vi "opencvSegmentMultiple.vi"(6 "maxYInStack":dbl, 7 "maxXInStack":dbl, 8 "ImgIn":u16[][][](array[numeric])) -> (0 "NeuronN[last frame]":u16, 1 "maxY":dbl, 2 "NeuronXY[last frame]":u16[](array[numeric]), 3 "NeuronN[frame]":u16[](array[numeric]), 4 "maxX":dbl, 5 "NeuronXY[frame]":u16[][](array[numeric]))   [LabVIEW 2017]
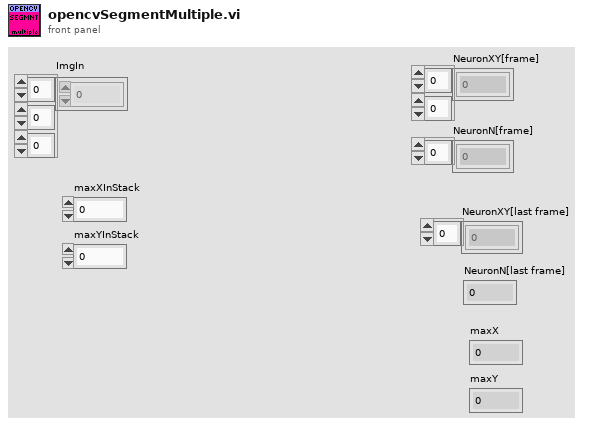
[diagram p1: front panel]
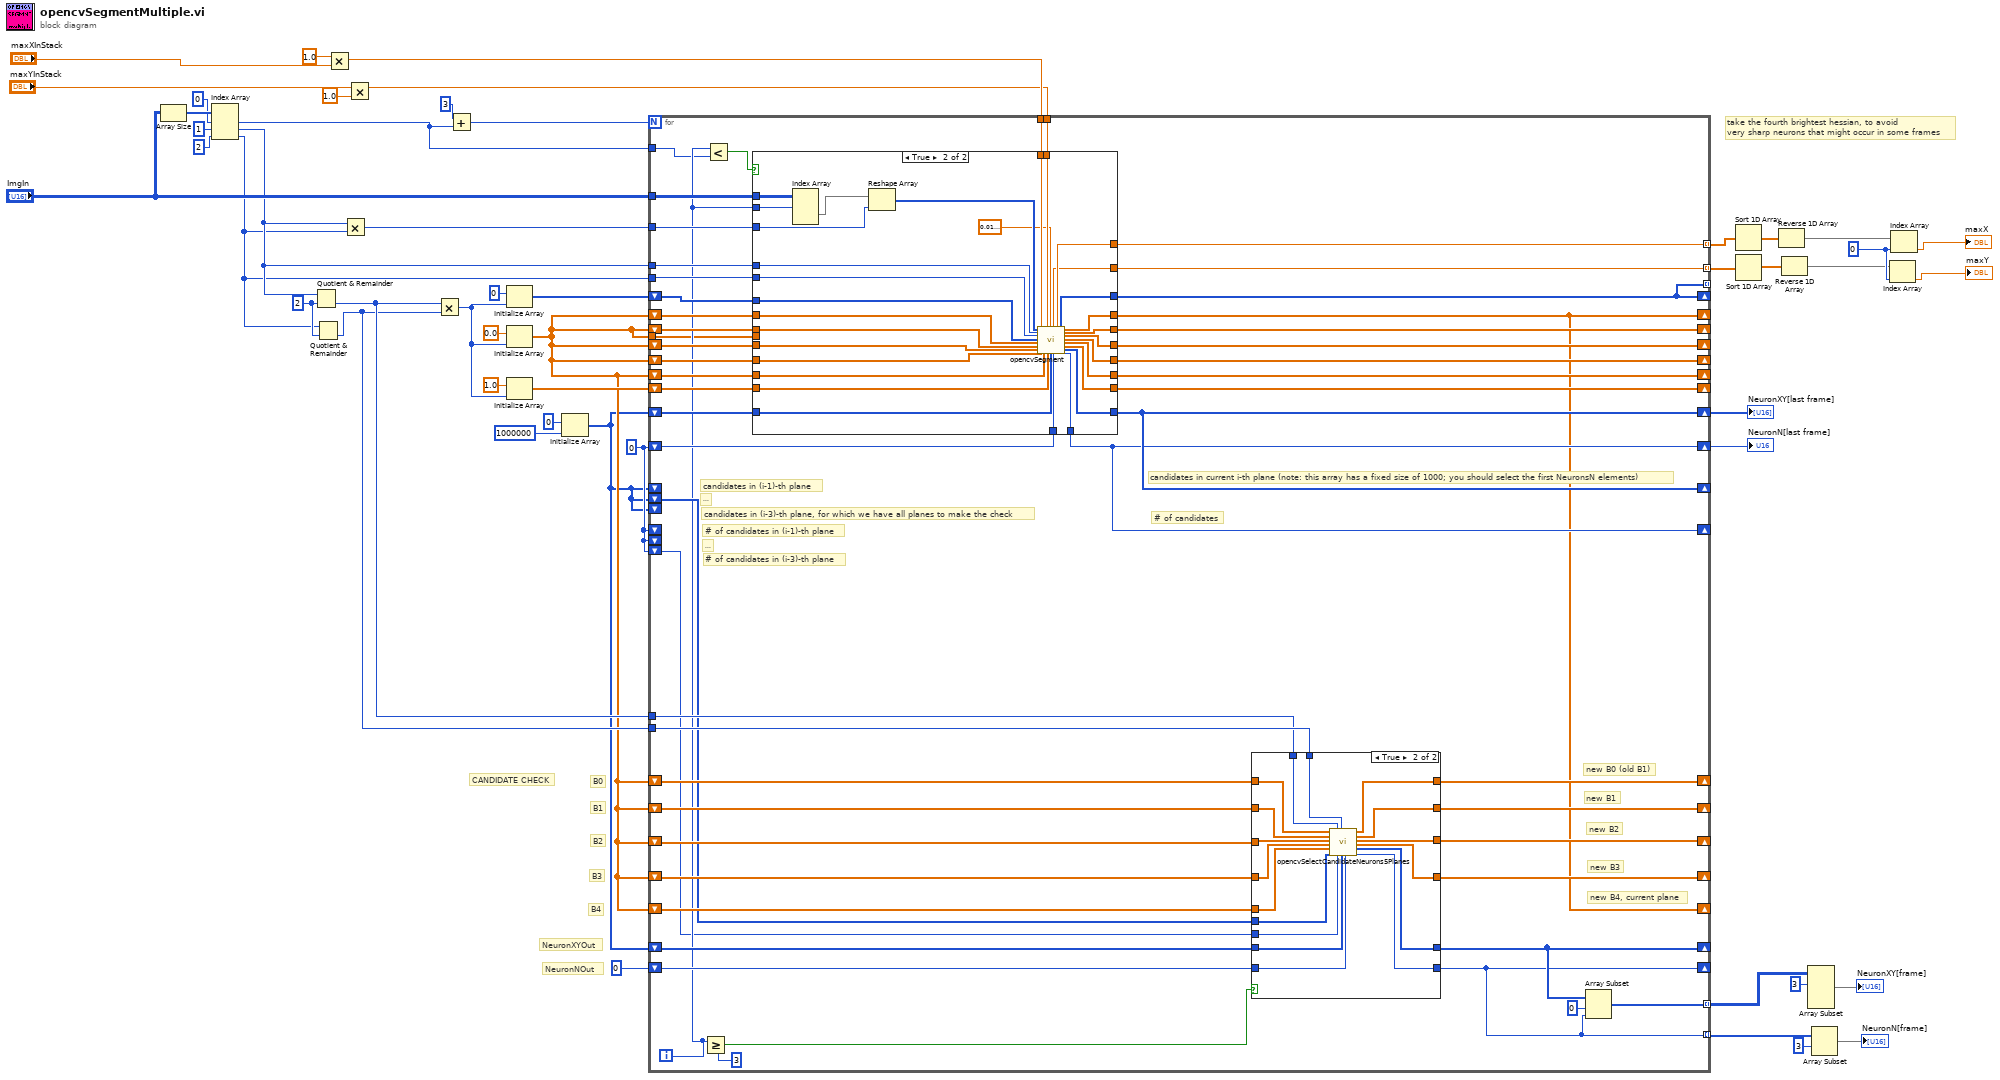
[diagram p0: block diagram]
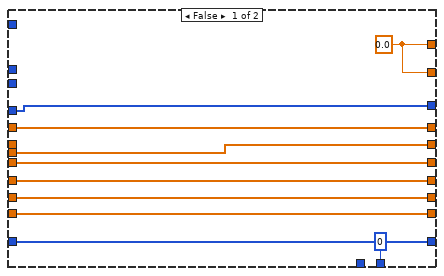
[diagram p2: hidden frame]
diagram:
  w3 = 0 ("y")
  w37 = 2 ("y")
  w11 = u16 0
  # "take the fourth brightest hessian, to avoid\nvery sharp neurons that might occur in some frames"
  # "NeuronNOut"
  # "NeuronXYOut"
  # "B4"
  # "B3"
  # "B2"
  # "B1"
  # "B0"
  # "CANDIDATE CHECK"
  n1 = Array Size(array="ImgIn") -> (size(s)=w49:i32[])
  n2 = Index Array(array=w49, index #1=0 ("index"), index #2=1 ("index"), index #3=2 ("index")) -> (element #1=w6:i32, element #2=w35:i32, element #3=w34:i32)
  n3 = Quotient & Remainder(x=w35, y=w37) -> (floor(x/y)=w32:i32)  [unwired: 1 out]
  n4 = Quotient & Remainder(x=w34, y=w37) -> (floor(x/y)=w31:i32)  [unwired: 1 out]
  n5 = Multiply(x=1.0, y="maxXInStack") -> (x*y=w25:dbl)
  n6 = Multiply(x=w35, y=w34) -> (x*y=w33:i32)
  n7 = Multiply(x="maxYInStack", y=1.0) -> (x*y=w23:dbl)
  n8 = Multiply(x=w32, y=w31) -> (x*y=w36:i32)
  n9 = Add(x=3, y=w6) -> (x+y=w18:i32)
  n10 = Initialize Array(u16 0 ("element"), w36) -> (w43:u16[])
  n11 = Initialize Array(sgl 0.0 ("element"), w36) -> (w13:sgl[])
  n12 = Initialize Array(sgl 1.0 ("element"), w36) -> (w42:sgl[])
  n13 = Initialize Array(u16 0 ("element"), 1000000 ("dimension size")) -> (w10:u16[])
  n14 = for {
    N: w18 -> [_]
    tunnel: "ImgIn" -> [w60]
    shift-right: [w50] -> _
    shift-left: w43 -> [w98]
    shift-right: [w52] -> _
    shift-left: w13 -> [w97]
    shift-right: [w53] -> _
    shift-left: w13 -> [w96]
    shift-right: [w63] -> _
    shift-left: w13 -> [w95]
    shift-right: [w62] -> _
    shift-left: w13 -> [w94]
    shift-right: [w61] -> _
    shift-left: w13 -> [w93]
    shift-right: [w88] -> _
    shift-left: w42 -> [w92]
    shift-right: [w72] -> w29
    shift-left: w10 -> [w91]
    shift-right: [w64] -> w28
    shift-left: w11 -> [w90]
    tunnel: w33 -> [w89]
    tunnel: w35 -> [w100]
    tunnel: w34 -> [w99]
    shift-right: [w77] -> _
    shift-left: w13 -> [w86]
    shift-right: [w76] -> _
    shift-left: w13 -> [w85]
    shift-right: [w75] -> _
    shift-left: w13 -> [w84]
    shift-right: [w74] -> _
    shift-left: w13 -> [w83]
    shift-right: [w52] -> _
    shift-left: w13 -> [w82]
    tunnel: w32 -> [w80]
    tunnel: w31 -> [w81]
    shift-right: [w73] -> _
    shift-left: w10 -> [w79]
    shift-right: [w55] -> _
    shift-left: u16 0 -> [w78]
    shift-right: [w72] -> _
    shift-left: w10 -> [_]
    shift-right: [w64] -> _
    shift-left: w11 -> [_]
    shift-left: w10 -> [w71]
    shift-left: w11 -> [_]
    tunnel: [w69] -> w9 mode=indexing
    tunnel: [w55] -> w16 mode=indexing
    tunnel: w25 -> [w68]
    tunnel: w23 -> [w67]
    tunnel: [w66] -> w21 mode=indexing
    tunnel: [w65] -> w7 mode=indexing
    tunnel: w6 -> [w58]
    tunnel: w13 -> [w54]
    shift-left: w11 -> [w51]
    shift-left: w10 -> [_]
    tunnel: [w50] -> _ mode=indexing
    i -> [w59]
    # "candidates in (i-3)-th plane, for which we have all planes to make the check"
    # "# of candidates in (i-3)-th plane"
    # "..."
    # "# of candidates in (i-1)-th plane"
    # "new B4, current plane"
    # "new B3"
    # "new B2"
    # "new B1"
    # "new B0 (old B1)"
    # "# of candidates"
    # "..."
    # "candidates in (i-1)-th plane"
    # "candidates in current i-th plane (note: this array has a fixed size of 1000; you should select the first NeuronsN elements)"
    n15 = Greater Or Equal?(x=w59, y=3) -> (x >= y?=w56:bool)
    n16 = Less?(x=w59, y=w58) -> (x < y?=w57:bool)
    n17 = case shown="True" w57 {
      tunnel: w100 -> [_ w140]
      tunnel: w99 -> [_ w139]
      tunnel: w98 -> [w109 w138]
      tunnel: w97 -> [w108 w137]
      tunnel: w96 -> [_ w136]
      tunnel: w95 -> [w107 w135]
      tunnel: w94 -> [w106 w134]
      tunnel: w93 -> [w105 w133]
      tunnel: w92 -> [w104 w132]
      tunnel: w91 -> [w103 w131]
      tunnel: w90 -> [_ w130]
      tunnel: w89 -> [_ w129]
      tunnel: [w104 w128] -> w88
      tunnel: [w103 w127] -> w72
      tunnel: w68 -> [_ w125]
      tunnel: w67 -> [_ w124]
      tunnel: [w110 w123] -> w66
      tunnel: [w110 w122] -> w65
      tunnel: [u16 0 ("NeuronN Out") w121] -> w64
      tunnel: [w101 w120] -> w53
      tunnel: [w107 w119] -> w63
      tunnel: [w106 w118] -> w62
      tunnel: [w105 w117] -> w61
      tunnel: [w109 w116] -> w50
      tunnel: [w108 w115] -> w52
      tunnel: w60 -> [_ w114]
      tunnel: w59 -> [_ w112]
      tunnel: w54 -> [w101 _]
      frame False {
        w110 = 0.0 ("maxX")
      }
      frame True {
        n18 = Index Array(array=w114, index (dim 0)=w112) -> (element=w113:u16[][])  [unwired: 2 in]
        n19 = Reshape Array(w113, w129) -> (w126:u16[])
        n20 = call "opencvSegment.vi"("ImgIn"=w126, "sizex"=w140, "sizey"=w139, "ArrA"=w138, "ArrB"=w137, "ArrBX"=w136, "ArrBY"=w135, "ArrBth"=w134, "maxXInStack"=w125, "ArrBdil"=w133, "maxYInStack"=w124, "ArrUno"=w132, "threshold"=sgl 0.02, "NeuronXY"=w131, "NeuronN"=w130) -> ("maxY"=w122:dbl, "maxX"=w123:dbl, "ArrA Out"=w116:u16[], "ArrB Out"=w115:sgl[], "ArrBX Out"=w120:sgl[], "ArrBY Out"=w119:sgl[], "ArrBth Out"=w118:sgl[], "ArrBdil Out"=w117:sgl[], "ArrUno Out"=w128:sgl[], "NeuronXY Out"=w127:u16[], "NeuronN Out"=w121:u16)  [unwired: 2 in]
      }
    }
    n21 = case shown="True" w56 {
      tunnel: w86 -> [_ w163]
      tunnel: w85 -> [w146 w162]
      tunnel: w84 -> [w145 w161]
      tunnel: w83 -> [w144 w160]
      tunnel: w82 -> [w143 w159]
      tunnel: w81 -> [_ w147]
      tunnel: w80 -> [_ w158]
      tunnel: w79 -> [w142 w157]
      tunnel: w78 -> [w141 w156]
      tunnel: [w146 w155] -> w77
      tunnel: [w145 w154] -> w76
      tunnel: [w144 w153] -> w75
      tunnel: [w143 w152] -> w74
      tunnel: [w142 w151] -> w73
      tunnel: [w141 w150] -> w55
      tunnel: w51 -> [_ w149]
      tunnel: w71 -> [_ w148]
      frame False {
      }
      frame True {
        n22 = call "opencvSelectCandidateNeurons5Planes.vi"("ArrB0"=w163, "ArrB1"=w162, "ArrB2"=w161, "ArrB3"=w160, "ArrB4"=w159, "NeuronXYin"=w148, "sizeBx"=w158, "NeuronNin"=w149, "sizeBy"=w147, "NeuronXYout"=w157, "NeuronNout"=w156) -> ("ArrB1 out"=w155:sgl[], "ArrB2 out"=w154:sgl[], "ArrB3 out"=w153:sgl[], "ArrB4 out"=w152:sgl[], "NeuronXYout out"=w151:u16[], "NeuronNout out"=w150:u16)  [unwired: 3 in]
      }
    }
    n23 = Array Subset(array=w73, index=0, length=w55) -> (w69:u16[])
  }
  "NeuronXY[last frame]" <- w29
  "NeuronN[last frame]" <- w28
  n24 = Sort 1D Array(array=w21) -> (sorted array=w5:dbl[])
  n25 = Sort 1D Array(array=w7) -> (sorted array=w2:dbl[])
  n26 = Reverse 1D Array(array=w5) -> (reversed array=w4:dbl[])
  n27 = Reverse 1D Array(array=w2) -> (reversed array=w1:dbl[])
  n28 = Array Subset(array=w9, index (row)=3 ("index")) -> (→"NeuronXY[frame]":u16[][])  [unwired: 3 in]
  n29 = Array Subset(array=w16, index=3) -> (→"NeuronN[frame]":u16[])  [unwired: 1 in]
  n30 = Index Array(array=w1, index=w3) -> (element=→"maxY":dbl)
  n31 = Index Array(array=w4, index=w3) -> (element=→"maxX":dbl)
